vi "Get PS Status.vi"(8 "error in (no error)":errorcluster, 10 "Status":variant, 11 "PS Driver AMI4xx.lvlib:PS Driver AMI4xx.lvclass":refnum<class "PS Driver AMI4xx.lvclass">) -> (0 "error out":errorcluster, 2 "Status out":variant, 3 "PS Driver AMI4xx.lvlib:PS Driver AMI4xx.lvclass out":refnum<class "PS Driver AMI4xx.lvclass">)   [LabVIEW 2021, in "PS Driver.lvlib" / "PS Driver AMI4xx.lvclass"]
uses:
  PS Driver AMI4xx.lvclass
  PS Driver with Persistence.lvclass
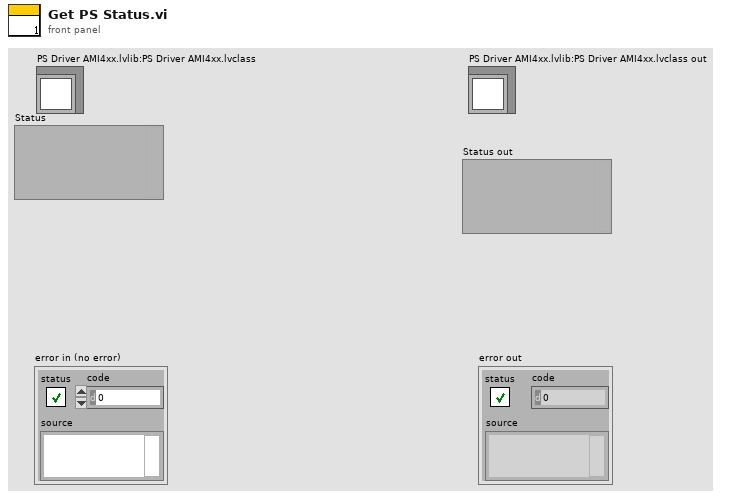
[diagram p1: front panel]
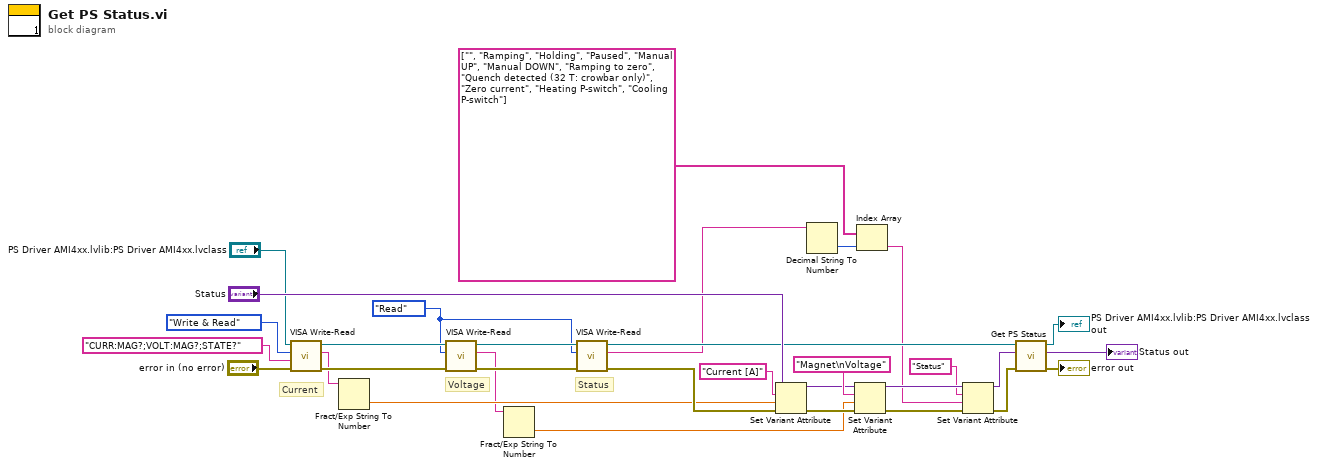
[diagram p0: block diagram]
diagram:
  w17 = enum16{"Write", "Read", "Write & Read"}."Read" ("Action")
  # "Status"
  # "Voltage"
  # "Current"
  n1 = call "VISA Write-Read.vi"("error in (no error)"="error in (no error)", "Command String"="CURR:MAG?;VOLT:MAG?;STATE?", "Action"=enum16{"Write", "Read", "Write & Read"}."Write & Read", "PS Driver.lvlib:PS Driver AMI4xx.lvclass"="PS Driver AMI4xx.lvlib:PS Driver AMI4xx.lvclass") -> ("error out"=w22:errorcluster, "Response string"=w4:string, "PS Driver.lvlib:PS Driver AMI4xx.lvclass out"=w23:refnum<class "PS Driver AMI4xx.lvclass">)  [unwired: 4 in, 1 out]
  n2 = Fract/Exp String To Number(string=w4) -> (number=w3:dbl)  [unwired: 3 in, 1 out]
  n3 = call "VISA Write-Read.vi"("error in (no error)"=w22, "Action"=w17, "PS Driver.lvlib:PS Driver AMI4xx.lvclass"=w23) -> ("error out"=w18:errorcluster, "Response string"=w2:string, "PS Driver.lvlib:PS Driver AMI4xx.lvclass out"=w20:refnum<class "PS Driver AMI4xx.lvclass">)  [unwired: 5 in, 1 out]
  n4 = Fract/Exp String To Number(string=w2) -> (number=w1:dbl)  [unwired: 3 in, 1 out]
  n5 = call "VISA Write-Read.vi"("error in (no error)"=w18, "Action"=w17, "PS Driver.lvlib:PS Driver AMI4xx.lvclass"=w20) -> ("error out"=w5:errorcluster, "Response string"=w6:string, "PS Driver.lvlib:PS Driver AMI4xx.lvclass out"=w19:refnum<class "PS Driver AMI4xx.lvclass">)  [unwired: 5 in, 1 out]
  n6 = Set Variant Attribute(Variant="Status", name="Current [A]", value=w3, error in=w5) -> (Variant out=w25:variant, error out=w27:errorcluster)  [unwired: 1 out]
  n7 = Decimal String To Number(string=w6) -> (number=w11:i32)  [unwired: 2 in, 1 out]
  n8 = Set Variant Attribute(Variant=w25, name="Magnet\nVoltage", value=w1, error in=w27) -> (Variant out=w14:variant, error out=w15:errorcluster)  [unwired: 1 out]
  n9 = Index Array(array=string[] ["", "Ramping", "Holding", "Paused", "Manual UP", "Manual DOWN", "Ramping to zero", "Quench detected (32 T: crowbar only)", "Zero current", "Heating P-switch", "Cooling P-switch"], index=w11) -> (element=w9:string)
  n10 = Set Variant Attribute(Variant=w14, name="Status", value=w9, error in=w15) -> (Variant out=w12:variant, error out=w7:errorcluster)  [unwired: 1 out]
  n11 = call-parent "Get PS Status.vi"("error in (no error)"=w7, "Status"=w12, "PS Driver.lvlib:PS Driver.lvclass"=w19) -> ("error out"=→"error out":errorcluster, "Status out"=→"Status out":variant, "PS Driver.lvlib:PS Driver.lvclass out"=→"PS Driver AMI4xx.lvlib:PS Driver AMI4xx.lvclass out":refnum<class "PS Driver AMI4xx.lvclass">)  [unwired: 6 in]
